vi "Dequeue.vi"(8 "error in (no error)":errorcluster, 9 "timeout (ms) (Default = -1)":i32=-1) -> (0 "error out":errorcluster, 2 "Data":variant, 3 "Command":T1=enum."Shutdown Module")   [LabVIEW 2022 SP3]
doc: "Receives a command and feeds it to the module Message Handling Loop (MHL)."
uses:
  Command.ctl
panel:
  # "Development\ncontrols/indicators useful for development and testing, but which are not outputs of the VI"
  # "Input\nInputs to the VI"
  # "Output\nOutputs of the VI"
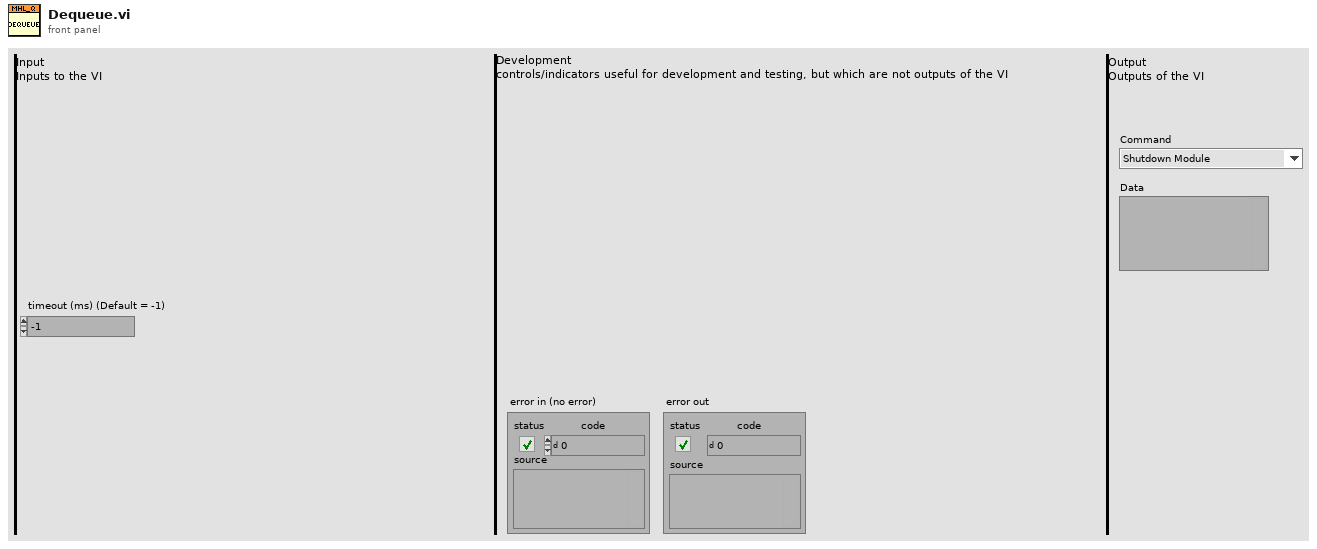
[diagram p1: front panel]
types:
  T1 = typedef "Command.ctl" = enum16{"Init Module", "Shutdown Module", "Local Error Handler", "Init Tickboxes", "Handle Value Change - Add to Project", "Handle Value Change - Add to Owner", "Handle Value Change - Add to Virtual Folder"}
  T2 = typedef "Message.ctl" = cluster{"Command":T1, "Data":variant}
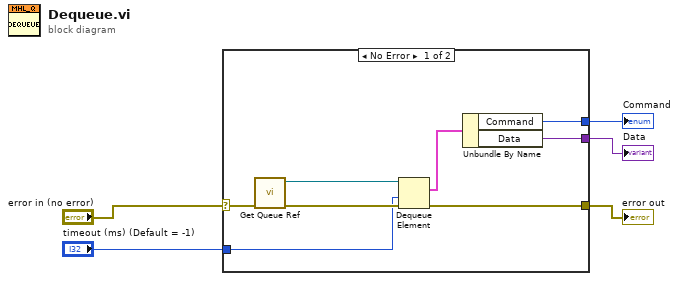
[diagram p0: block diagram]
diagram:
  n1 = case shown="No Error" "error in (no error)" {
    selector: "error in (no error)" -> [w13 w14]
    tunnel: [w11 w14] -> w4
    tunnel: "timeout (ms) (Default = -1)" -> [w9 _]
    tunnel: [w7 _] -> w2
    tunnel: [w6 _] -> w1
    frame No Error {
      n2 = call "Get Queue Ref.vi"("error in (no error)"=w13) -> ("error out"=w12:errorcluster, "Queue Ref"=w10:refnum<queue>)  [unwired: 9 in]
      n3 = Dequeue Element(queue=w10, timeout in ms (-1)=w9, error in (no error)=w12) -> (element=w8:T2, error out=w11:errorcluster)  [unwired: 2 out]
      n4 = Unbundle By Name(w8) -> ("Command"=w7:T1, "Data"=w6:variant)
    }
    frame Error {
    }
  }
  "error out" <- w4
  "Command" <- w2
  "Data" <- w1
